vi "SetGXMLHdr.vi"(8 "error in (no error)":errorcluster, 10 "ChanHdr":T1, 11 "Channel in":refnum<class "Channel.lvclass">) -> (0 "error out":errorcluster, 3 "Channel out":refnum<class "Channel.lvclass">)   [LabVIEW 2018, in "Measurement Channels.lvlib" / "Channel.lvclass"]
uses:
  Channel.lvclass
  ChanProps_TD.ctl
  Channel.lvclass/Channel.ctl
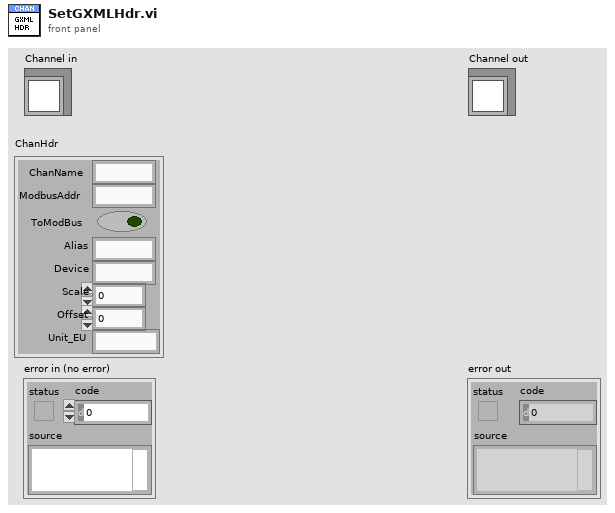
[diagram p1: front panel]
types:
  T1 = typedef "Measurement Channels.lvlib/Channel.lvclass/ChanProps_TD.ctl" = cluster{"ChanName":string, "ModbusAddr":string, "ToModBus":bool, "Alias":string, "Device":string, "Unit_EU":string, "Scale":dbl, "Offset":dbl}
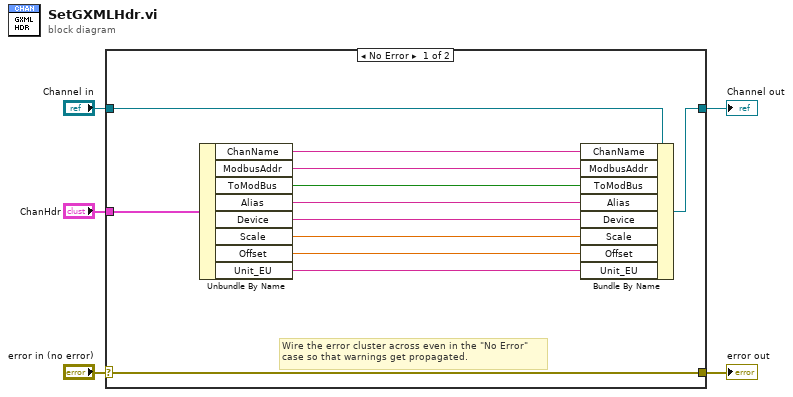
[diagram p0: block diagram]
diagram:
  n1 = case shown="No Error" "error in (no error)" {
    selector: "error in (no error)" -> [w17 w19]
    tunnel: [w17 w19] -> w4
    tunnel: [w6 w18] -> w2
    tunnel: "Channel in" -> [w7 w18]
    tunnel: "ChanHdr" -> [w8 _]
    frame No Error {
      # "Wire the error cluster across even in the \"No Error\"\ncase so that warnings get propagated."
      n2 = Unbundle By Name(w8) -> ("ChanName"=w16:string, "ModbusAddr"=w15:string, "ToModBus"=w14:bool, "Alias"=w13:string, "Device"=w12:string, "Scale"=w11:dbl, "Offset"=w10:dbl, "Unit_EU"=w9:string)
      n3 = Bundle By Name(cluster=w7, "ChanName"=w16, "ModbusAddr"=w15, "ToModBus"=w14, "Alias"=w13, "Device"=w12, "Scale"=w11, "Offset"=w10, "Unit_EU"=w9) -> (w6:refnum<class "Channel.lvclass">)
    }
    frame Error {
    }
  }
  "error out" <- w4
  "Channel out" <- w2
